vi "toggleCtlVis.vi"(8 "error in (no error)":errorcluster, 9 "ctlarr":T1, 10 "Variant":variant, 11 "tag?":string) -> (0 "error out":errorcluster, 1 "ctlarrOut":T1)   [LabVIEW 2017]
uses:
  RefArray/RefArray.ctl
panel:
  in  "element":cluster{"tab?":string, "newState?":bool}
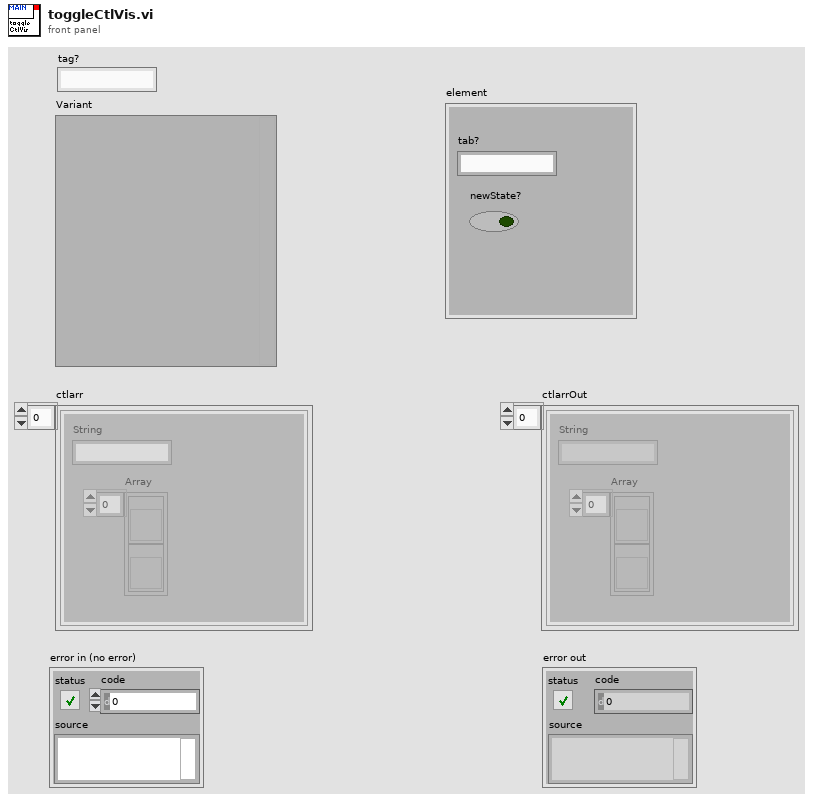
[diagram p1: front panel]
types:
  T1 = typedef "RefArray.ctl" = cluster{"String":string, "Array":refnum<vi>[]}[]
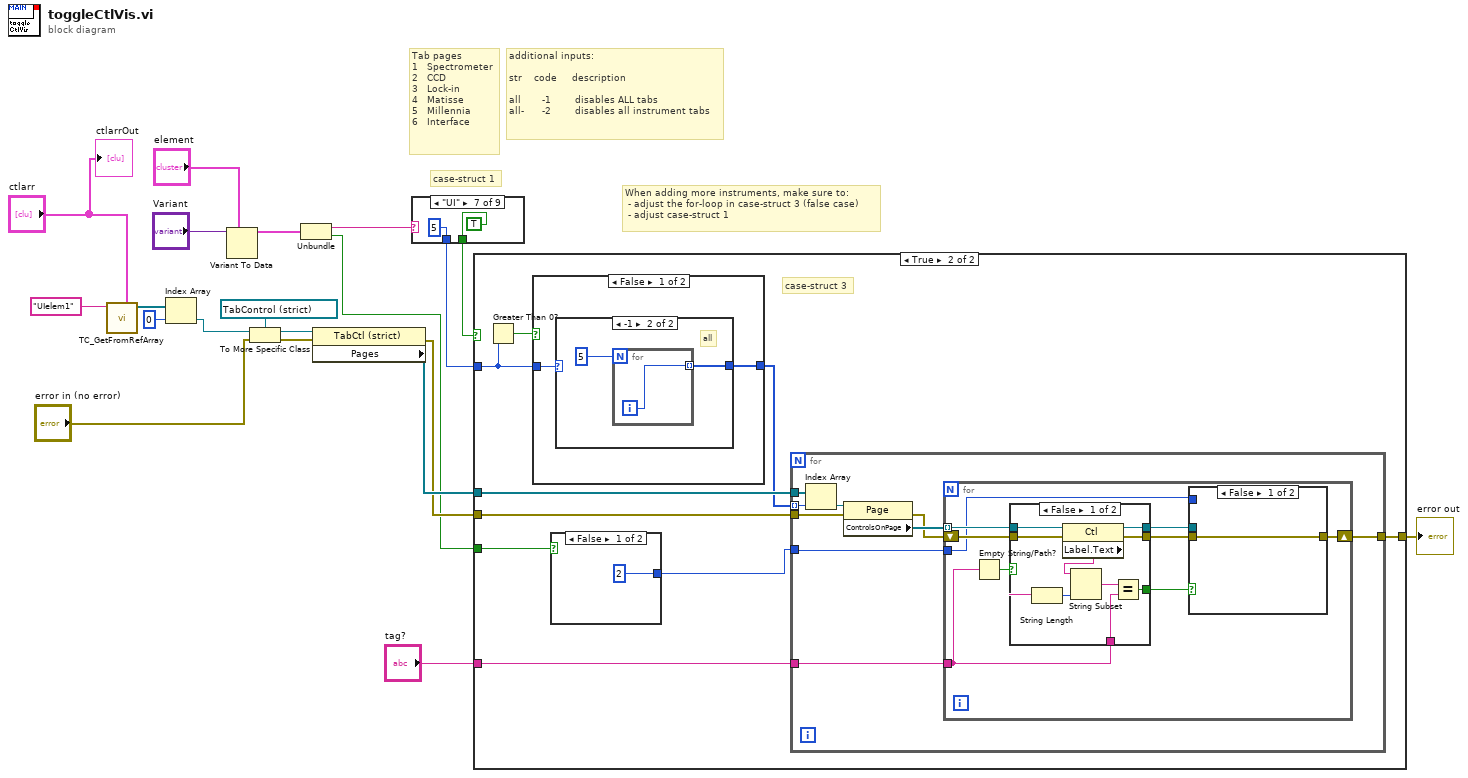
[diagram p0: block diagram]
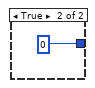
[diagram p3: hidden frame]
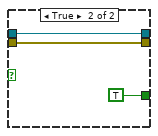
[diagram p4: hidden frame]
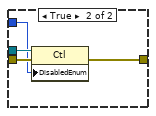
[diagram p5: hidden frame]
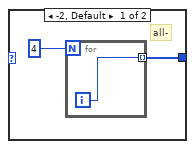
[diagram p6: hidden frame]
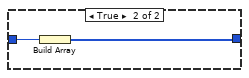
[diagram p7: hidden frame]
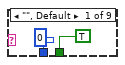
[diagram p8: hidden frame]
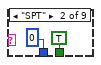
[diagram p9: hidden frame]
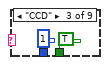
[diagram p10: hidden frame]
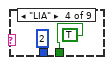
[diagram p11: hidden frame]
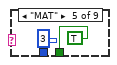
[diagram p12: hidden frame]
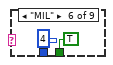
[diagram p13: hidden frame]
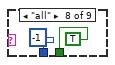
[diagram p14: hidden frame]
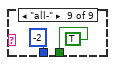
[diagram p15: hidden frame]
diagram:
  # "case-struct 1"
  # "When adding more instruments, make sure to:\n - adjust the for-loop in case-struct 3 (false case)\n - adjust case-struct 1"
  # "additional inputs:\n\nstr    code     description\n\nall       -1        disables ALL tabs\nall-      -2        disables all instrument tabs"
  # "Tab pages\n1   Spectrometer\n2   CCD\n3   Lock-in\n4   Matisse\n5   Millennia\n6   Interface"
  n1 = call "TC_GetFromRefArray.vi"("arrayIn"="ctlarr", "NameToFind"="UIelem1") -> ("refArray"=w16:refnum<vi>[])  [unwired: 8 in, 1 out]
  n2 = Index Array(array=w16, index=0) -> (element=w14:refnum<vi>)
  n3 = Variant To Data(type="element", Variant="Variant") -> (data=w18:cluster{"tab?":string, "newState?":bool})  [unwired: 1 in, 1 out]
  n4 = To More Specific Class(target class=refnum<vi> refnum ("Settings"), reference=w14, error in="error in (no error)") -> (specific class reference=w12:refnum<vi>, error out=w11:errorcluster)
  n5 = Unbundle(w18) -> ("tab?"=w9:string, "newState?"=w5:bool)
  n6 = property class="TabCtl (strict)"(reference=w12, error in=w11) -> (error out=w6:errorcluster, "Pages"=w10:refnum<vi>[])  [unwired: 1 out]
  n7 = case shown="\"UI\"" w9 {
    tunnel: [0 0 1 2 3 4 5 -1 -2] -> w8
    tunnel: [TRUE TRUE TRUE TRUE TRUE TRUE TRUE TRUE TRUE] -> w7
    frame "", Default {
    }
    frame "SPT" {
    }
    frame "CCD" {
    }
    frame "LIA" {
    }
    frame "MAT" {
    }
    frame "MIL" {
    }
    frame "UI" {
    }
    frame "all" {
    }
    frame "all-" {
    }
  }
  n8 = case shown="True" w7 {
    tunnel: w10 -> [_ w44]
    tunnel: w8 -> [_ w46]
    tunnel: w6 -> [_ w45]
    tunnel: w5 -> [_ w42]
    tunnel: [_ w40] -> w4
    tunnel: "tag?" -> [_ w39]
    frame False {
    }
    frame True {
      # "case-struct 3"
      n9 = Greater Than 0?(x=w46) -> (x > 0?=w47:bool)
      n10 = case shown="False" w47 {
        tunnel: w46 -> [w86 w94]
        tunnel: [w85 w93] -> w43
        frame False {
          n11 = case shown="-1" w86 {
            tunnel: [w88 w91] -> w85
            frame -2, Default {
              # "all-"
              n12 = for {
                N: 4 -> [_]
                tunnel: [w89] -> w88 mode=indexing
                i -> [w89]
              }
            }
            frame -1 {
              # "all"
              n13 = for {
                N: 5 -> [_]
                tunnel: [w92] -> w91 mode=indexing
                i -> [w92]
              }
            }
          }
        }
        frame True {
          n14 = Build Array(w94) -> (w93:i32[])
        }
      }
      n15 = case shown="False" w42 {
        tunnel: [2 0] -> w41
        frame False {
        }
        frame True {
        }
      }
      n16 = for {
        tunnel: w45 -> [w57]
        tunnel: w44 -> [w56]
        tunnel: w43 -> [w55] mode=indexing
        tunnel: w41 -> [w52]
        tunnel: [w51] -> w40
        tunnel: w39 -> [w50]
        n17 = Index Array(array=w56, index=w55) -> (element=w58:refnum<vi>)
        n18 = property class="Page"(reference=w58, error in=w57) -> (error out=w53:errorcluster, "ControlsOnPage"=w54:refnum<vi>[])  [unwired: 1 out]
        n19 = for {
          tunnel: w54 -> [w67] mode=indexing
          shift-right: [w62] -> w51
          shift-left: w53 -> [w66]
          tunnel: w52 -> [w61]
          tunnel: w50 -> [w60]
          n20 = Empty String/Path?(string/path=w60) -> (empty?=w59:bool)
          n21 = case shown="False" w59 {
            tunnel: w67 -> [w76 w79]
            tunnel: w66 -> [w75 w78]
            tunnel: [w74 w79] -> w65
            tunnel: [w73 w78] -> w64
            tunnel: [w70 TRUE] -> w63
            tunnel: w60 -> [w69 _]
            frame False {
              n22 = String Length(string=w69) -> (length=w68:i32)
              n23 = property class="Ctl"(reference=w76, error in=w75) -> (reference out=w74:refnum<vi>, error out=w73:errorcluster, "Label.Text"=w71:string)
              n24 = String Subset(string=w71, length (rest)=w68) -> (substring=w72:string)  [unwired: 1 in]
              n25 = Equal?(x=w72, y=w69) -> (x = y?=w70:bool)
            }
            frame True {
            }
          }
          n26 = case shown="False" w63 {
            tunnel: w65 -> [_ w84]
            tunnel: w64 -> [w80 w83]
            tunnel: [w80 w82] -> w62
            tunnel: w61 -> [_ w81]
            frame False {
            }
            frame True {
              n27 = property class="Ctl"(reference=w84, error in=w83, "DisabledEnum"=w81) -> (error out=w82:errorcluster)  [unwired: 1 out]
            }
          }
        }
      }
    }
  }
  "error out" <- w4
  "ctlarrOut" <- "ctlarr"
